vi "calcdelaySD.vi"(2 "current point":i32, 3 "timedelays":dbl[](array[numeric])) -> (0 "Delay, mm":dbl)   [LabVIEW 2015]
uses:
  globalVarSD.vi
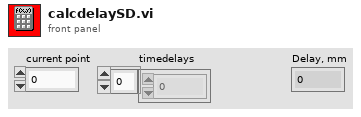
[diagram p1: front panel]
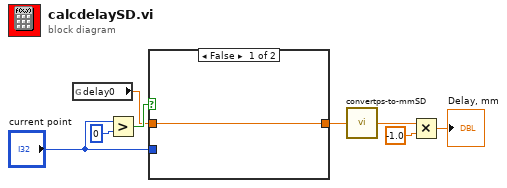
[diagram p0: block diagram]
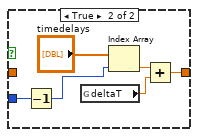
[diagram p2: hidden frame]
diagram:
  n1 = global read "globalVarSD.vi" "delay0"() -> (w6:dbl)
  n2 = Greater?(x="current point", y=0) -> (0:w7:bool)
  n3 = case shown="False" w7 {
    tunnel: [w9 w12] -> w1
    tunnel: w6 -> [w9 _]
    tunnel: "current point" -> [_ w11]
    frame False {
    }
    frame True {
      n4 = Decrement(x=w11) -> (x-1=w10:i32)
      n5 = global read "globalVarSD.vi" "deltaT"() -> (w13:dbl)
      n6 = Index Array(array="timedelays", index=w10) -> (element=w14:dbl)
      n7 = Add(x=w14, y=w13) -> (x+y=w12:dbl)
    }
  }
  n8 = call "convertps-to-mmSD.vi"("ps"=w1) -> ("mm"=w4:dbl)
  n9 = Multiply(x=w4, y=-1.0) -> (x*y=→"Delay, mm":dbl)
